vi "RPOP.vi"(0 "TCP session out":refnum<k5>, 1 "Key":string, 11 "error in":errorcluster) -> (4 "TCP session out":refnum<k5>, 6 "Data":T1, 15 "error out":errorcluster)   [LabVIEW 2023]
uses:
  SubVIs/Controls/redis-data.ctl
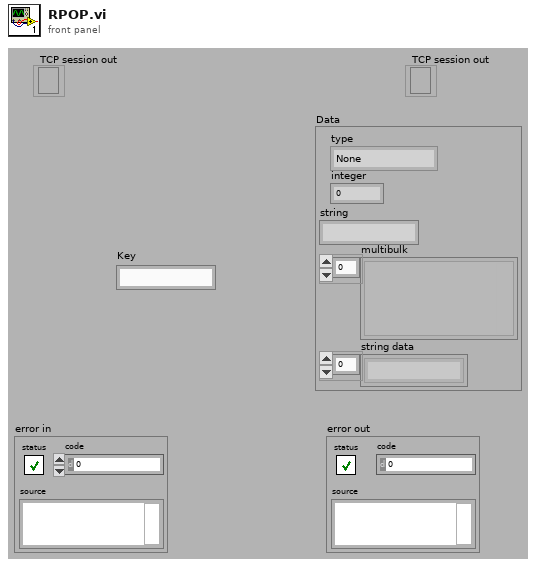
[diagram p1: front panel]
types:
  T1 = typedef "redis-data.ctl" = cluster{"type":enum16{"None", "Error", "Status", "Nil", "Integer", "String", "Multibulk"}, "integer":i64, "string":string, "multibulk":variant[], "string data":string[]}
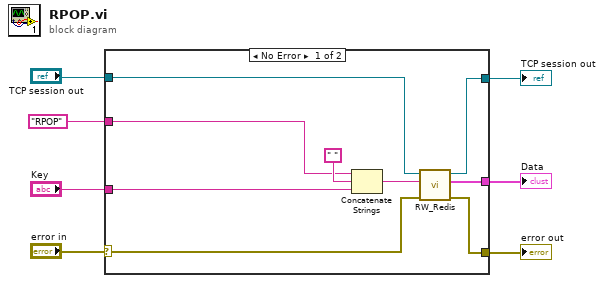
[diagram p0: block diagram]
diagram:
  n1 = case shown="No Error" "error in" {
    selector: "error in" -> [w13 w18]
    tunnel: "Key" -> [w10 _]
    tunnel: "RPOP" -> [w15 _]
    tunnel: "TCP session out" -> [w9 w17]
    tunnel: [w12 w18] -> w5
    tunnel: [w11 _] -> w1
    tunnel: [w8 w17] -> w2
    frame No Error {
      n2 = Concatenate Strings(w15, " ", w10) -> (w14:string)
      n3 = call "RW_Redis.vi"("error in"=w13, "command"=w14, "TCP session in"=w9) -> ("error out"=w12:errorcluster, "Data"=w11:T1, "TCP session out"=w8:refnum<k5>)  [unwired: 6 in]
    }
    frame Error {
    }
  }
  "error out" <- w5
  "TCP session out" <- w2
  "Data" <- w1
